vi "Init Queue Array.vi"(8 "error in (no error)":errorcluster, 10 "element":T1, 11 "Array in":string[](array[string])) -> (0 "error out":errorcluster, 3 "Array out":refnum<queue>[](array[refnum]))   [LabVIEW 2017]
uses:
  Queue Element.ctl
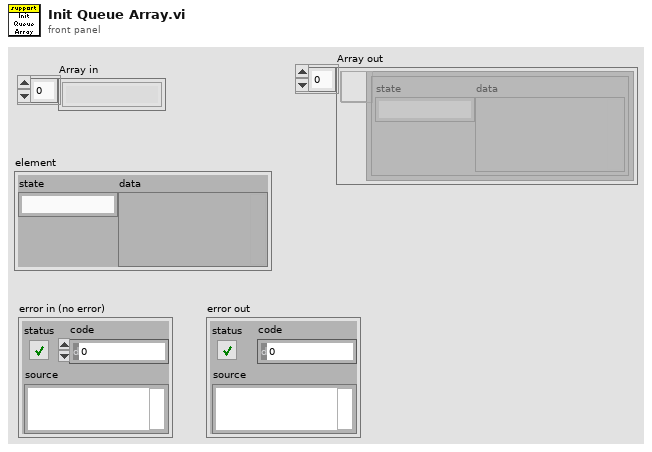
[diagram p1: front panel]
types:
  T1 = typedef "Queue Element.ctl" = cluster{"state":string, "data":variant}
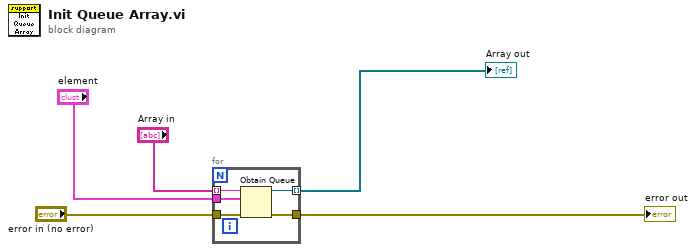
[diagram p0: block diagram]
diagram:
  n1 = for {
    tunnel: "element" -> [w10]
    tunnel: "error in (no error)" -> [w9]
    tunnel: [w8] -> w3
    tunnel: "Array in" -> [w7] mode=indexing
    tunnel: [w6] -> w5 mode=indexing
    n2 = Obtain Queue(name (unnamed)=w7, element data type=w10, error in (no error)=w9) -> (queue out=w6:refnum<queue>, error out=w8:errorcluster)  [unwired: 2 in, 1 out]
  }
  "Array out" <- w5
  "error out" <- w3
